vi "Read Message Icon.vi"(11 "Message Scripter in":refnum<class "Message Scripter.lvclass">) -> (2 "Message Icon":refnum<class "Icon.lvclass">)   [LabVIEW 2020, in "Message Maker.lvlib" / "Message Scripter.lvclass"]
uses:
  Message Scripter.lvclass
  <vilib>/LabVIEW Icon API/lv_icon/Classes/Icon/Icon.lvclass
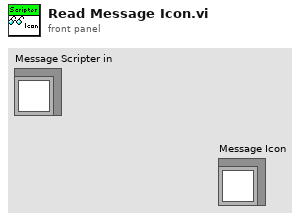
[diagram p1: front panel]
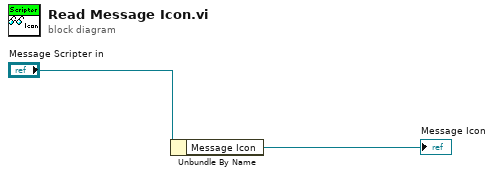
[diagram p0: block diagram]
diagram:
  n1 = Unbundle By Name("Message Scripter in") -> ("Message Icon"=→"Message Icon":refnum<class "Icon.lvclass">)
